vi "TxDatos-1.vi"() -> ()   [LabVIEW 2020]
uses:
  <vilib>/httpClient/PUTBuffer.vi
  <vilib>/httpClient/LabVIEWHTTPClient.lvlib
panel:
  in  "Accionamiento":dbl(knob) scale=0.0..10.0
  in  "Rele":bool
  in  "stop":bool
  out "error PUT":errorcluster
  out "body PUT":string
  out "headers PUT":string
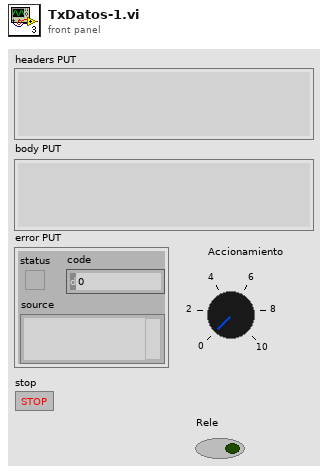
[diagram p1: front panel]
types:
  T1 = cluster{"Accionamiento":dbl, "Hora":string, "Data":string, "Rele":bool}
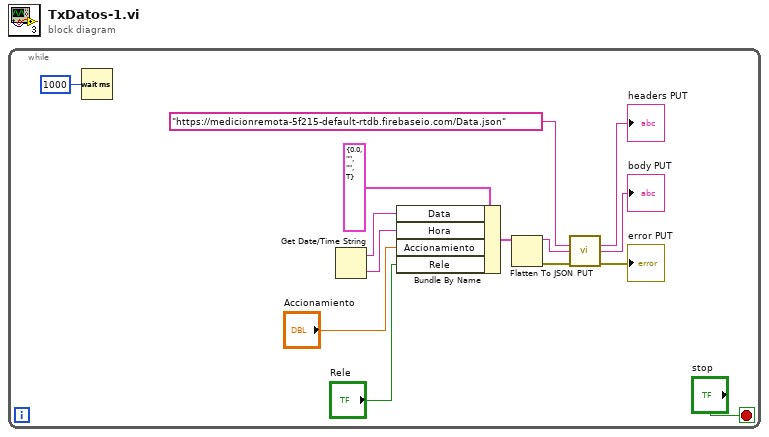
[diagram p0: block diagram]
diagram:
  n1 = while {
    stop <- "stop" stop-if-true
    n2 = Wait (ms)(milliseconds to wait=u32 1000) -> ()  [unwired: 1 out]
    n3 = Get Date/Time String() -> (date string=w2:string, time string=w1:string)  [unwired: 3 in]
    n4 = Bundle By Name(cluster=T1 {"Accionamiento"=0.0, "Hora"="", "Data"="", "Rele"=TRUE} ("output cluster"), "Data"=w2, "Hora"=w1, "Accionamiento"="Accionamiento", "Rele"="Rele") -> (w6:T1)
    n5 = Flatten To JSON(anything=w6) -> (JSON string=w13:string, 11:w12:errorcluster)  [unwired: 2 in]
    n6 = call-poly <vilib>:"PUT.vi"("url"="https://medicionremota-5f215-default-rtdb.firebaseio.com/Data.json", "buffer"=w13, "error in (no error)"=w12) -> ("headers"=→"headers PUT":string, "body"=→"body PUT":string, "error out"=→"error PUT":errorcluster)  [unwired: 9 in, 1 out]
  }
